vi "PI_Control_with_Anti_Windup_Sim.vi"(1 "Tr":dbl=1.0 min=1.0 step=1.0, 2 "bsp":dbl, 3 "ki":dbl, 4 "kp":dbl, 5 "y":dbl, 6 "r":dbl) -> (0 "u":dbl)   [LabVIEW 2010]
doc: "Proportional-integral (PI) controller."
uses:
  <vilib>/Simulation/Implementation/Shared/SIMSCR Execution Mode.ctl
  <vilib>/Simulation/Scripting/Companion Diagram/SimConfigNode/SimDog.xnode
  <vilib>/Simulation/Scripting/Companion Diagram/SimConfigNode/SimParams.ctl
  <vilib>/Simulation/Scripting/Companion Diagram/SimConfigNode/_simSolvers.ctl
  <vilib>/Simulation/Implementation/Shared/SIM block execution type.ctl
  <vilib>/Simulation/Implementation/Shared/SIM limit type.ctl
  <vilib>/Simulation/Implementation/Shared/SIM trigger type.ctl
  <vilib>/Simulation/Implementation/XNodeFramework/SimXNode/SimX.xnode
  <vilib>/Simulation/Nonlinear/Implementation/NILVSim Saturation.llb/SIM Saturation (scalar).vi
  <vilib>/Simulation/SignalArithmetic/Implementation/NILVSim Gain.llb/SIM Gain (scalar).vi
  <vilib>/Simulation/ContinuousLinear/Implementation/NILVSim Integrator new.llb/SIM Integrator distributor (scalar).vi
  <vilib>/Simulation/ContinuousLinear/Implementation/NILVSim Integrator new.llb/SIM Integrator collector (scalar).vi
  <vilib>/Simulation/Utility/Implementation/NILVSim Memory.llb/NILVSim Memory (core).vi
  <vilib>/Simulation/Implementation/Shared/NILVSim_Manager.vi
  <vilib>/Simulation/Implementation/Shared/NILVSim_GetModelError.vi
  <vilib>/Simulation/Implementation/Shared/NILVSim_FinalizeModel.vi
  <vilib>/Simulation/Implementation/Shared/NILVSim_GetSimErrorInfo.vi
  <vilib>/Simulation/Implementation/Shared/NILVSim_GenerateString.vi
  <vilib>/Simulation/Implementation/Shared/NILVSim_GetBlockNameAndCallChain.vi
  <vilib>/Simulation/Implementation/Shared/NILVSim_GetSimErrorString.vi
  <vilib>/Simulation/Implementation/Shared/NILVSim_GetBlockNameAndCallChainSizes.vi
  <vilib>/Simulation/Implementation/Shared/NILVSim_GetBlockNameAndCallChain Core.vi
  <vilib>/Simulation/Implementation/Shared/SIM Unbundle Sim Info.vi
  <vilib>/Simulation/Implementation/Shared/SIM SimErrorHandler.vi
  <vilib>/Simulation/Implementation/Shared/SIM Bundle Sim Info.vi
  <vilib>/Simulation/Implementation/Shared/NILVSim_Initialize.vi
  <vilib>/dlg_ctls.llb/Space Constant.vi
  <vilib>/Simulation/ContinuousLinear/Implementation/NILVSim Integrator new.llb/SIM Integrator (scalar).vi
  <vilib>/Simulation/Implementation/Shared/NI_SIM_Implementation.lvlib
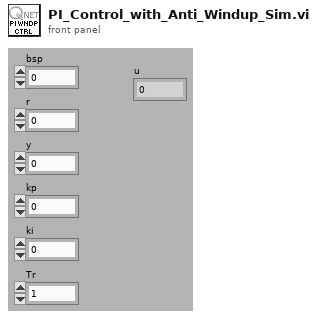
[diagram p1: front panel]
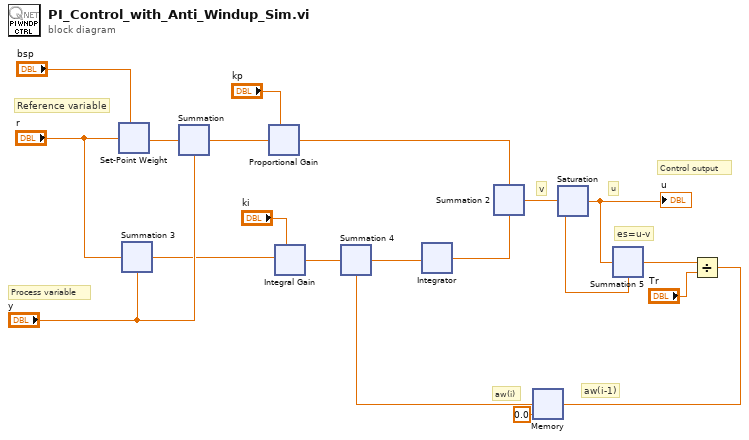
[diagram p0: block diagram]
diagram:
  # "aw(i)"
  # "aw(i-1)"
  # "es=u-v"
  # "v"
  # "u"
  # "Control output"
  # "Process variable"
  # "Reference variable"
  n1 = xnode "Set-Point Weight"("gain"="bsp", "input"="r") -> ("output"=w5:dbl)  [unwired: 2 in]
  n2 = xnode ("Summation 3")("Operand1"="r", "Operand2"="y") -> ("Result"=w8:dbl)
  n3 = xnode ("Summation")("Operand1"=w5, "Operand2"="y") -> ("Result"=w16:dbl)
  n4 = xnode "Proportional Gain"("gain"="kp", "input"=w16) -> ("output"=w17:dbl)  [unwired: 2 in]
  n5 = xnode "Integral Gain"("gain"="ki", "input"=w8) -> ("output"=w7:dbl)  [unwired: 2 in]
  n6 = xnode ("Summation 4")("Operand1"=w7, "Operand2"=w11) -> ("Result"=w9:dbl)
  n7 = xnode ("Integrator")("input"=w9) -> ("output"=w13:dbl)  [unwired: 1 in, 2 out]
  n8 = xnode ("Summation 2")("Operand1"=w17, "Operand2"=w13) -> ("Result"=w2:dbl)
  n9 = xnode ("Saturation")("input"=w2) -> ("output"=w3:dbl)  [unwired: 2 in]
  "u" <- w3
  n10 = xnode ("Summation 5")("Operand1"=w3, "Operand2"=w2) -> ("Result"=w14:dbl)
  n11 = Divide(x=w14, y="Tr") -> (x/y=w10:dbl)
  n12 = xnode ("Memory")("input"=w10, "initial value"=0.0) -> ("output"=w11:dbl)  [unwired: 1 in]
